vi "ROTPEN MPC template.vi"() -> ()   [LabVIEW 2018]
uses:
  <vilib>/Simulation/Implementation/XNodeFramework/SimXNode/SimX.xnode
  <vilib>/Simulation/Scripting/Companion Diagram/SimConfigNode/SimDog.xnode
  <vilib>/Simulation/ContinuousLinear/Implementation/NILVSim Transfer Function Direct.llb/SIM Transfer Function Direct (SISO).vi
  <vilib>/Simulation/SignalArithmetic/Implementation/NILVSim Gain.llb/SIM Gain (scalar).vi
  <vilib>/Quanser/Rapid Control Prototyping Toolkit/hardware/HIL Immediate IO/CL HIL Write.vi
  <vilib>/Quanser/Rapid Control Prototyping Toolkit/hardware/HIL Immediate IO/CL HIL Read.vi
  <vilib>/Simulation/Implementation/Shared/SIMSCR Execution Mode.ctl
  <vilib>/Simulation/Scripting/Companion Diagram/SimConfigNode/_simSolvers.ctl
  <vilib>/Simulation/Scripting/Companion Diagram/SimConfigNode/SimParams.ctl
  <vilib>/Simulation/DataSources/Implementation/NILVSim Signal Generator.llb/SIM Signal Generator (scalar).vi
  <vilib>/Simulation/Utility/Implementation/SIM Halt.vi
  <vilib>/Quanser/Rapid Control Prototyping Toolkit/hardware/HIL Immediate IO/_TypeSpecific/CL HIL Read Encoder (Vector).vi
  <vilib>/Simulation/Nonlinear/Implementation/NILVSim Saturation.llb/SIM Saturation (scalar).vi
  <vilib>/Quanser/Rapid Control Prototyping Toolkit/hardware/HIL Immediate IO/_TypeSpecific/CL HIL Write Analog (Scalar).vi
  <vilib>/imath/engines/lvmath2/RunTimeEngine/IndexRead/NIMS M(S,S).vi
  <vilib>/imath/engines/lvmath2/RunTimeEngine/IndexRead/NIMS V(S).vi
  <vilib>/imath/engines/lvmath2/RunTimeEngine/IndexReplace/NIMS M(S,S)=S.vi
  <vilib>/imath/engines/lvmath2/RunTimeEngine/ErrorHandling/NIMS_Create Error From Enums.vi
  <vilib>/imath/engines/lvmath/Plug In/Control Design/BuiltInFunctions/ss/NIMS_CD_ss(A,B,C,D).vi
  <vilib>/imath/engines/lvmath/Plug In/Control Design/BuiltInFunctions/c_to_d/NIMS_CD_c_to_d(SS,TS,STR,DBL).vi
  <vilib>/imath/engines/lvmath2/RunTimeEngine/NodeEndStatement/NIMS_NodeEndStatement_Output.vi
  <vilib>/imath/engines/lvmath2/RunTimeEngine/ErrorHandling/NIMS_Finalize Error.vi
  <vilib>/imath/engines/lvmath2/RunTimeEngine/IndexRead/NIMS V(R2).vi
  <vilib>/imath/engines/lvmath2/RunTimeEngine/BuiltInFunctions/diag/NIMS_diag.vi
  <vilib>/imathl/engines/lvmath/Functions/Error Handling/Create Error.vi
  <vilib>/imath/engines/lvmath2/RunTimeEngine/ArithmeticOperatorToken/NIMS_ArithmeticOperator_multmx.vi
  <vilib>/imath/engines/lvmath2/RunTimeEngine/ArithmeticOperatorToken/NIMS_ArithmeticOperator_plus.vi
  <vilib>/imath/engines/lvmath2/RunTimeEngine/BuiltInFunctions/eye/NIMS_M=eye(I32, I32).vi
  <vilib>/imath/engines/lvmath2/RunTimeEngine/IndexReplace/NIMS M(R2,$)=M.vi
  <vilib>/imath/engines/lvmath2/RunTimeEngine/RangeToken/NIMS_Range_R2 - Integer.vi
  <vilib>/imath/engines/lvmath2/RunTimeEngine/CommandStatement/MC_CommandStatement_break.vi
  <vilib>/imath/engines/lvmath2/RunTimeEngine/ArithmeticOperatorToken/NIMS_ArithmeticOperator_powermx(M,M).vi
  <vilib>/imath/engines/lvmath2/RunTimeEngine/MatrixToken/NIMS_MatrixToken_M_M.vi
  <vilib>/imath/engines/lvmath2/RunTimeEngine/IndexReplace/NIMS M(R2,R2)=M.vi
  <vilib>/imath/engines/lvmath2/RunTimeEngine/RowToken/NIMS_RowToken_M_M.vi
  <vilib>/addons/Control Design/_Model Construction/NI_LinSys_Model Information.lvlib
  <vilib>/addons/Control Design/_Model Construction/Model Information.llb/Model Information SubVIs/cd_Get Matrices From SS Model.vi
  <vilib>/imath/engines/lvmath2/RunTimeEngine/BuiltInFunctions/fmin_qp/NIMS_fmin_qp.vi
  <vilib>/imath/engines/lvmath2/RunTimeSupport/NIMS_Complex To Real.vi
  <vilib>/imath/engines/lvmath2/RunTimeSupport/NIMS_Get Any Vector_w Error - Matrix.vi
  <vilib>/imath/engines/lvmath2/RunTimeEngine/ArithmeticOperatorToken/NIMS_ArithmeticOperator_multmx(M,CV).vi
panel:
  in  "weight O4":dbl
  in  "weight O3":dbl
  in  "weight I1":dbl
  in  "weight O2":dbl
  in  "weight O1":dbl
  in  "Control Horizon (Nc)":u64 step=1
  in  "Prediction Horizon (Np)":u64 step=1
  in  "stop":bool
  out "Motor Voltage (V)":dbl(graph)
  out "Rotary Arm Position (deg)":cluster{"output":dbl, "output":dbl}(graph)
  out "Pendulum Angle (deg)":dbl(graph)
  in  "Frequency (Hz)":dbl(slide)=0.2 min=0.0 max=0.5 step=0.05 scale=0.0..0.5 scale format="%#_3f"
  in  "Amplitude (deg)":dbl(slide) min=0.0 max=40.0 step=5.0 scale=0.0..40.0
  # "MPC Control Experiment"
  # "Rotary Arm Reference Signal"
  # "MPC Parameters"
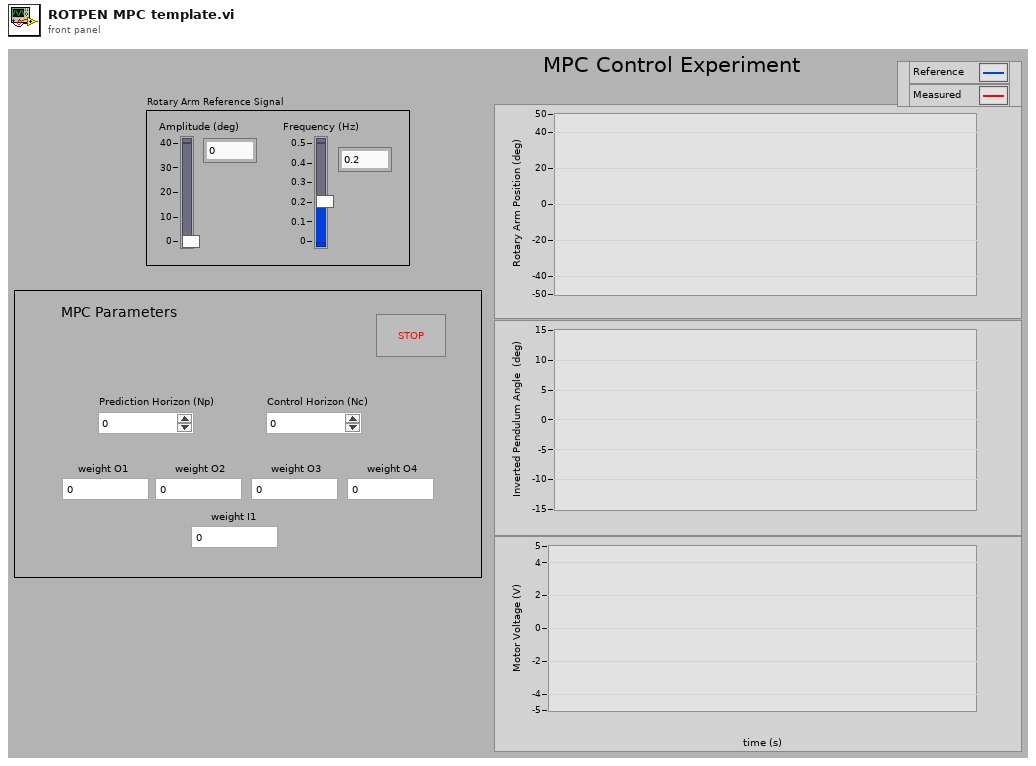
[diagram p1: front panel]
types:
  T1 = typedef "NI_LinSys_Model Typedefs.lvlib/CD State Space Model (MIMO).ctl" = cluster{"properties":T2, "A":dbl[][], "B":dbl[][], "C":dbl[][], "D":dbl[][], "StateNames":string[], "Transport Delay":dbl[][]}
  T2 = typedef "NI_LinSys_Model Typedefs.lvlib/CD General Elements.ctl" = cluster{"Model name":string, "Input names":string[], "Output names":string[], "Input Delays":dbl[], "Output Delays":dbl[], "Sampling Time":dbl, "Notes":string}
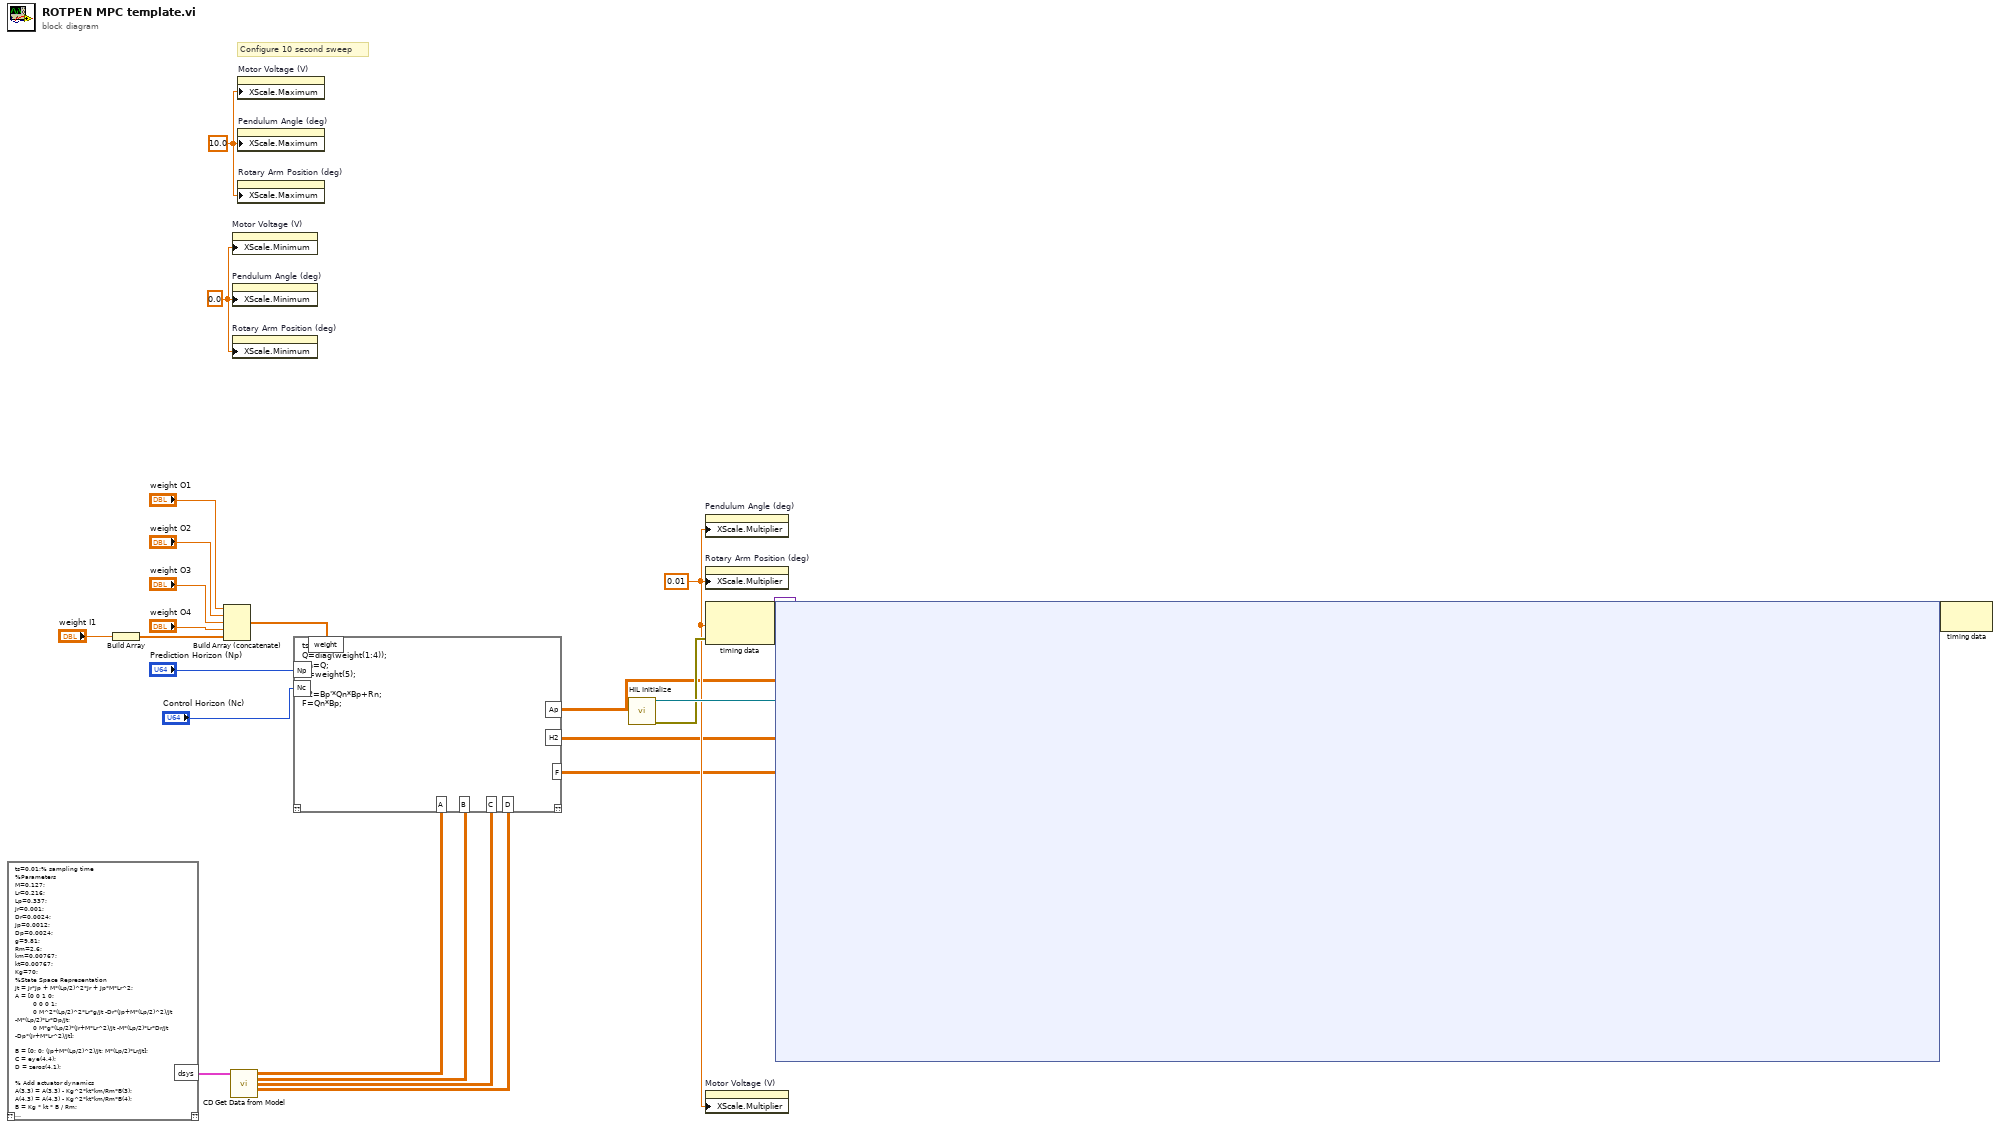
[diagram p0: block diagram]
diagram:
  w19 = 0.0 ("X Scale.Range:Maximum")
  w18 = 10.0 ("X Scale.Range:Maximum")
  w20 = 0.01 ("Step Size (s)")
  # "Configure 10 second sweep"
  n1 = mathscript code="ts=0.01;% sampling time\n%Parameters\nM=0.127;\nLr=0.216;\nLp=0.337;\nJr=0.001;\nDr=0.0024;\nJp=0.0012;\nDp=0.0024;\ng=9.81;\nRm=2.6;\nkm=0.00767;\nkt=0.00767;\nKg=70;\n%State Space Representation\nJt = Jr*Jp + M*(Lp/2)^2*Jr + Jp*M*Lr^2;\nA = [0 0 1 0;\n         0 0 0 1;\n         0 M^2*(Lp/2)^2*Lr*g/Jt -Dr*(Jp+M*(Lp/2)^2)/Jt -M*(Lp/2)*Lr*Dp/Jt;\n         0 M*g*(Lp/2)*(Jr+M*Lr^2)/Jt -M*(Lp/2)*Lr*Dr/Jt -Dp*(Jr+M*Lr^2)/Jt];\n\nB = [0; 0; (Jp+M*(Lp/2)^2)/Jt; M*(Lp/2)*Lr/Jt];\nC = eye(4,4);\nD = zeros(4,1);\n\n% Add actuator dynamics\nA(3,3) = A(3,3) - Kg^2*kt*km/Rm*B(3);\nA(4,3) = A(4,3) - Kg^2*kt*km/Rm*B(4);\nB = Kg * kt * B / Rm;\n\nsys = ss(A,B,C,D);\ndsys=c2d(sys,ts);"() -> ("dsys"=w8:T1)  [unwired: 1 in, 1 out]
  n2 = Build Array ("Build Array 4")("weight I1") -> (w12:dbl[])
  n3 = Build Array (concatenate) ("Build Array 3")("weight O1", "weight O2", "weight O3", "weight O4", w12) -> (w11:dbl[])
  n4 = call-poly <vilib>:"CD Get Data from Model.vi"("State-Space Model"=w8) -> ("Matrix A"=w7:dbl[][], "Matrix B"=w6:dbl[][], "Matrix C"=w5:dbl[][], "Matrix D"=w4:dbl[][])  [unwired: 10 in, 1 out]
  n5 = property on="Motor Voltage (V)" class="WFChart (strict)"("XScale.Minimum"=w19) -> ()  [unwired: 2 in, 2 out]
  n6 = property on="Pendulum Angle (deg)" class="WFChart (strict)"("XScale.Minimum"=w19) -> ()  [unwired: 2 in, 2 out]
  n7 = property on="Rotary Arm Position (deg)" class="WFChart (strict)"("XScale.Minimum"=w19) -> ()  [unwired: 2 in, 2 out]
  n8 = property on="Motor Voltage (V)" class="WFChart (strict)"("XScale.Maximum"=w18) -> ()  [unwired: 2 in, 2 out]
  n9 = property on="Pendulum Angle (deg)" class="WFChart (strict)"("XScale.Maximum"=w18) -> ()  [unwired: 2 in, 2 out]
  n10 = property on="Rotary Arm Position (deg)" class="WFChart (strict)"("XScale.Maximum"=w18) -> ()  [unwired: 2 in, 2 out]
  n11 = mathscript code="ts=0.01;\nQ=diag(weight(1:4));\nQn=Q;\nR=weight(5);\n\nH2=Bp'*Qn*Bp+Rn;\nF=Qn*Bp;" ("MathScript Node 2")("Np"="Prediction Horizon (Np)", "Nc"="Control Horizon (Nc)", "weight"=w11, "A"=w7, "B"=w6, "C"=w5, "D"=w4) -> ("Ap"=w2:cdb[][], "F"=w1:cdb[][], "H2"=w3:cdb[][])  [unwired: 1 in, 1 out]
  n12 = call "HIL Initialize"() -> ("board out"=w22:refnum<class "HIL Board.lvclass">, "error out"=w21:errorcluster)  [unwired: 14 in]
  n13 = property on="Pendulum Angle (deg)" class="WFChart (strict)"("XScale.Multiplier"=w20) -> ()  [unwired: 2 in, 2 out]
  n14 = property on="Rotary Arm Position (deg)" class="WFChart (strict)"("XScale.Multiplier"=w20) -> ()  [unwired: 2 in, 2 out]
  n15 = node-c288(w20, w21) -> (w24:variant)
  n16 = property on="Motor Voltage (V)" class="WFChart (strict)"("XScale.Multiplier"=w20) -> ()  [unwired: 2 in, 2 out]
  n17 = node-c254 ("Control & Simulation Loop")(w24, w22, w3, w2, w1) -> (w23:variant)
  n18 = node-c288(w23) -> ()  [unwired: 1 out]
